vi "FTW-Actor-Destroy.vi"(0 "FTW Actor Instance":refnum<class "FTW-ActorExtended.lvclass">, 5 "Force Destroy?":bool=TRUE, 11 "error in":errorcluster) -> (15 "error out":errorcluster)   [LabVIEW 2013, in "FTW-ActorExtended.lvclass"]
uses:
  FTW-ActorExtended.lvclass
  Instance/FTW-ActorInstance.lvclass
  FTW-ActorExtended.lvclass/FTW-ActorExtended.ctl
  Connector/FTW-ActorConnector.lvclass
  Publisher/FTW-Publisher.lvclass
  Subscriber/FTW-Subscriber.lvclass
panel:
  # "Inputs"
  # "Outputs"
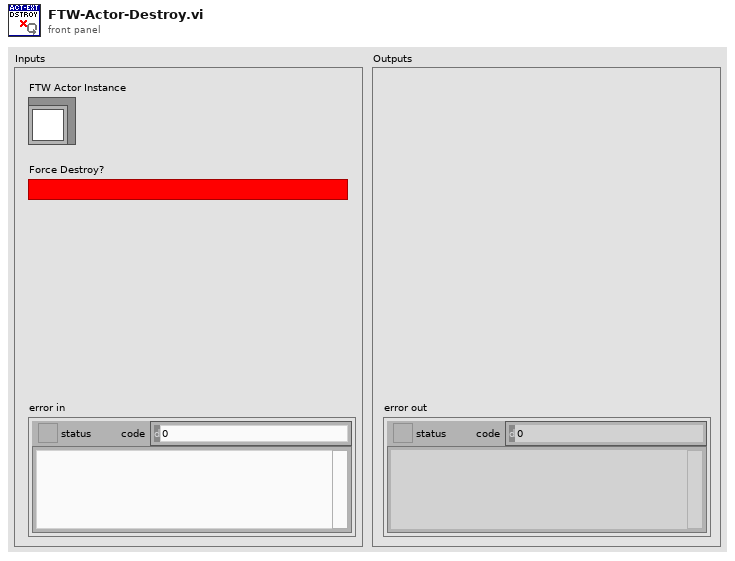
[diagram p1: front panel]
types:
  T1 = cluster{"Name":string, "URI":string, "Connector":refnum<class "FTW-ActorConnector.lvclass">}[]
  T2 = cluster{"Name":string, "URI":string, "Publisher":refnum<class "FTW-Publisher.lvclass">}[]
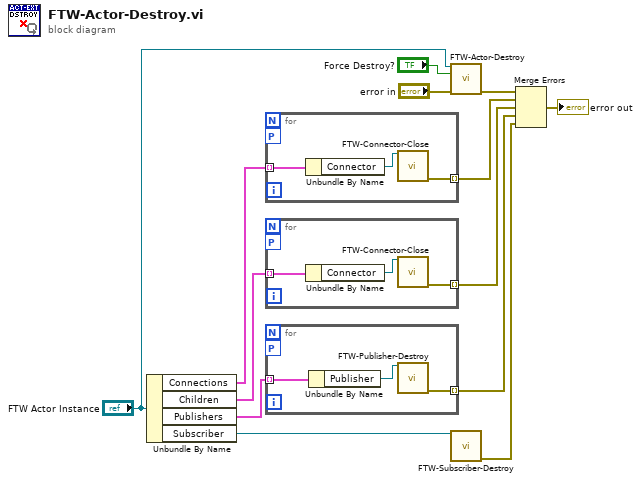
[diagram p0: block diagram]
diagram:
  n1 = Unbundle By Name("FTW Actor Instance") -> ("Connections"=w3:T1, "Children"=w1:T1, "Publishers"=w9:T2, "Subscriber"=w5:refnum<class "FTW-Subscriber.lvclass">)
  n2 = for {
    tunnel: [w16] -> w7 mode=indexing
    tunnel: w3 -> [w15] mode=indexing
    workers-P: _ -> [_]
    n3 = Unbundle By Name(w15) -> ("Connector"=w14:refnum<class "FTW-ActorConnector.lvclass">)
    n4 = call-dynamic "FTW-Connector-Close.vi"("FTW Actor Connector"=w14) -> ("error out"=w16:errorcluster)  [unwired: 14 in]
  }
  n5 = for {
    tunnel: [w19] -> w2 mode=indexing
    tunnel: w1 -> [w18] mode=indexing
    workers-P: _ -> [_]
    n6 = Unbundle By Name(w18) -> ("Connector"=w17:refnum<class "FTW-ActorConnector.lvclass">)
    n7 = call-dynamic "FTW-Connector-Close.vi"("FTW Actor Connector"=w17) -> ("error out"=w19:errorcluster)  [unwired: 14 in]
  }
  n8 = for {
    tunnel: [w22] -> w6 mode=indexing
    tunnel: w9 -> [w21] mode=indexing
    workers-P: _ -> [_]
    n9 = Unbundle By Name(w21) -> ("Publisher"=w20:refnum<class "FTW-Publisher.lvclass">)
    n10 = call "FTW-Publisher-Destroy.vi"("FTW-Publisher In"=w20) -> ("error out"=w22:errorcluster)  [unwired: 14 in]
  }
  n11 = call-parent "FTW-Actor-Destroy.vi"("FTW Actor Instance"="FTW Actor Instance", "Force Destroy?"="Force Destroy?", "error in"="error in") -> ("error out"=w8:errorcluster)  [unwired: 12 in]
  n12 = call "FTW-Subscriber-Destroy.vi"("FTW-Subscription In"=w5) -> ("error out"=w4:errorcluster)  [unwired: 14 in]
  n13 = Merge Errors(w8, w7, w2, w6, w4) -> (→"error out":errorcluster)
